vi "Draw.vi"(8 "error in (no error)":errorcluster, 10 "Picture in":picture, 11 "Line in":refnum<class "Line.lvclass">) -> (0 "error out":errorcluster, 2 "Picture out":picture, 3 "Line out":refnum<class "Line.lvclass">)   [LabVIEW 2015, in "Line.lvclass"]
uses:
  Line.lvclass
  Graphic/Graphic.lvclass/Graphic.ctl
  Graphic/Graphic.lvclass
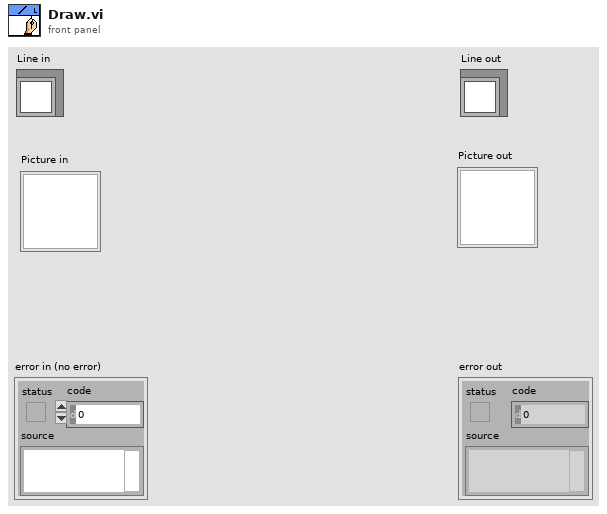
[diagram p1: front panel]
types:
  T1 = typedef "Graphic.lvclass/Style.ctl" = cluster{"Color":u32, "Pen":cluster{"Width":u16, "Style":enum32{"Solid", "Dash", "Dot", "DashDot", "DashDotDot"}}}
  T2 = cluster{"Width":u16, "Style":enum32{"Solid", "Dash", "Dot", "DashDot", "DashDotDot"}}
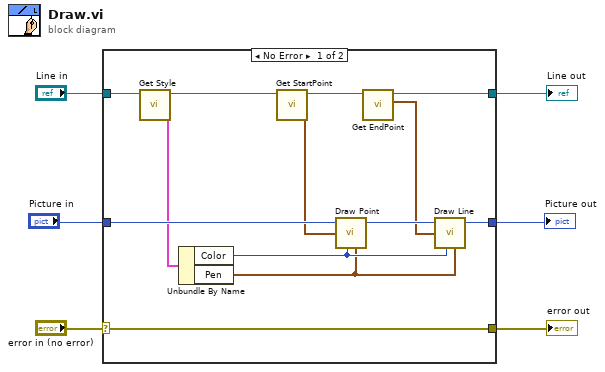
[diagram p0: block diagram]
diagram:
  n1 = case shown="No Error" "error in (no error)" {
    selector: "error in (no error)" -> [w19 w22]
    tunnel: "Line in" -> [w15 w21]
    tunnel: [w13 w21] -> w4
    tunnel: "Picture in" -> [w18 w20]
    tunnel: [w16 w20] -> w2
    tunnel: [w19 w22] -> w1
    frame No Error {
      n2 = call "Get Style.vi"("Graphic in"=w15) -> ("Style"=w9:T1, "Graphic out"=w10:refnum<class "Line.lvclass">)  [unwired: 8 in, 1 out]
      n3 = Unbundle By Name(w9) -> ("Color"=w8:u32, "Pen"=w7:T2)
      n4 = call "Get StartPoint.vi"("Graphic in"=w10) -> ("StartPoint"=w11:cluster{"x":i16, "y":i16}, "Graphic out"=w14:refnum<class "Line.lvclass">)  [unwired: 8 in, 1 out]
      n5 = call <vilib>:"Draw Point.vi"("picture"=w18, "point(x,y)"=w11, "color(black)"=w8, "pen"=w7) -> ("new picture"=w17:picture)  [unwired: 5 in]
      n6 = call "Get EndPoint.vi"("Graphic in"=w14) -> ("EndPoint"=w12:cluster{"x":i16, "y":i16}, "Graphic out"=w13:refnum<class "Line.lvclass">)  [unwired: 8 in, 1 out]
      n7 = call <vilib>:"Draw Line.vi"("picture"=w17, "end point"=w12, "color(black)"=w8, "pen"=w7) -> ("new picture"=w16:picture)  [unwired: 5 in]
    }
    frame Error {
    }
  }
  "error out" <- w1
  "Line out" <- w4
  "Picture out" <- w2
